vi "Update FIFO Address - 16-bit Address.vi"(0 "address in":u16, 5 "increment":bool, 7 "fifo depth":T1=10 items=["4"=2, "8"=3, "16"=4, "32"=5, "64"=6, "128"=7, "256"=8, "512"=9, "1024"=10, "2048"=11, "4096"=12, "8192"=13, "16384"=14, "32768"=15, "65536"=16]) -> (4 "address out":u16)   [LabVIEW 2011, in "FIFO.lvlib"]
uses:
  <instrlib>/RF-RIO/FIFO/FIFO/FPGA/FIFO.lvlib
  <instrlib>/RF-RIO/FIFO/FIFO/FPGA/Private/FIFO Depth - 16-bit Address.ctl
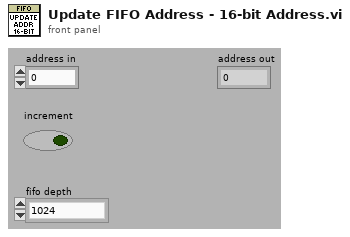
[diagram p1: front panel]
types:
  T1 = typedef "FIFO.lvlib/FIFO Depth - 16-bit Address.ctl" = u8
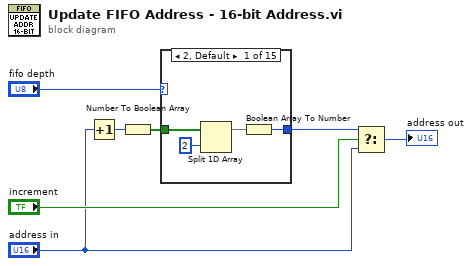
[diagram p0: block diagram]
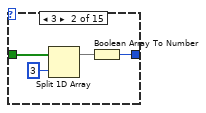
[diagram p2: hidden frame]
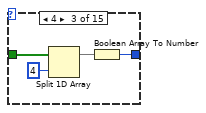
[diagram p3: hidden frame]
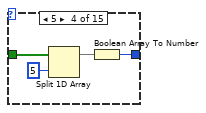
[diagram p4: hidden frame]
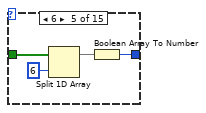
[diagram p5: hidden frame]
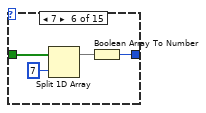
[diagram p6: hidden frame]
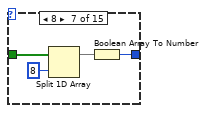
[diagram p7: hidden frame]
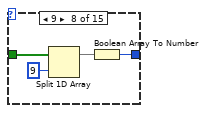
[diagram p8: hidden frame]
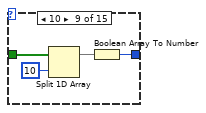
[diagram p9: hidden frame]
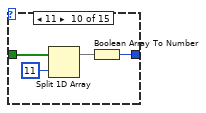
[diagram p10: hidden frame]
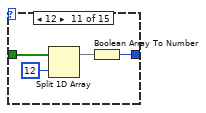
[diagram p11: hidden frame]
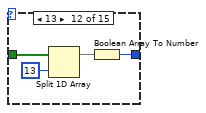
[diagram p12: hidden frame]
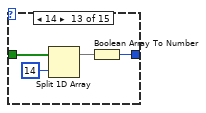
[diagram p13: hidden frame]
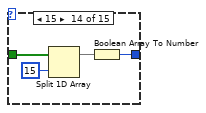
[diagram p14: hidden frame]
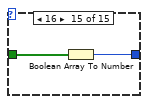
[diagram p15: hidden frame]
diagram:
  n1 = Increment(x="address in") -> (x+1=w2:u16)
  n2 = Number To Boolean Array(number=w2) -> (Boolean array=w1:bool[])
  n3 = case shown="2, Default" "fifo depth" {
    tunnel: w1 -> [w10 w14 w18 w22 w26 w30 w34 w38 w42 w46 w50 w54 w58 w62 w64]
    tunnel: [w11 w15 w19 w23 w27 w31 w35 w39 w43 w47 w51 w55 w59 w63 w65] -> w5
    frame 2, Default {
      n4 = Split 1D Array(array=w10, index=2) -> (first subarray=w8:bool[])  [unwired: 1 out]
      n5 = Boolean Array To Number(Boolean array=w8) -> (number=w11:u16)
    }
    frame 3 {
      n6 = Split 1D Array(array=w14, index=3) -> (first subarray=w12:bool[])  [unwired: 1 out]
      n7 = Boolean Array To Number(Boolean array=w12) -> (number=w15:u16)
    }
    frame 4 {
      n8 = Split 1D Array(array=w18, index=4) -> (first subarray=w16:bool[])  [unwired: 1 out]
      n9 = Boolean Array To Number(Boolean array=w16) -> (number=w19:u16)
    }
    frame 5 {
      n10 = Split 1D Array(array=w22, index=5) -> (first subarray=w20:bool[])  [unwired: 1 out]
      n11 = Boolean Array To Number(Boolean array=w20) -> (number=w23:u16)
    }
    frame 6 {
      n12 = Split 1D Array(array=w26, index=6) -> (first subarray=w24:bool[])  [unwired: 1 out]
      n13 = Boolean Array To Number(Boolean array=w24) -> (number=w27:u16)
    }
    frame 7 {
      n14 = Split 1D Array(array=w30, index=7) -> (first subarray=w28:bool[])  [unwired: 1 out]
      n15 = Boolean Array To Number(Boolean array=w28) -> (number=w31:u16)
    }
    frame 8 {
      n16 = Split 1D Array(array=w34, index=8) -> (first subarray=w32:bool[])  [unwired: 1 out]
      n17 = Boolean Array To Number(Boolean array=w32) -> (number=w35:u16)
    }
    frame 9 {
      n18 = Split 1D Array(array=w38, index=9) -> (first subarray=w36:bool[])  [unwired: 1 out]
      n19 = Boolean Array To Number(Boolean array=w36) -> (number=w39:u16)
    }
    frame 10 {
      n20 = Split 1D Array(array=w42, index=10) -> (first subarray=w40:bool[])  [unwired: 1 out]
      n21 = Boolean Array To Number(Boolean array=w40) -> (number=w43:u16)
    }
    frame 11 {
      n22 = Split 1D Array(array=w46, index=11) -> (first subarray=w44:bool[])  [unwired: 1 out]
      n23 = Boolean Array To Number(Boolean array=w44) -> (number=w47:u16)
    }
    frame 12 {
      n24 = Split 1D Array(array=w50, index=12) -> (first subarray=w48:bool[])  [unwired: 1 out]
      n25 = Boolean Array To Number(Boolean array=w48) -> (number=w51:u16)
    }
    frame 13 {
      n26 = Split 1D Array(array=w54, index=13) -> (first subarray=w52:bool[])  [unwired: 1 out]
      n27 = Boolean Array To Number(Boolean array=w52) -> (number=w55:u16)
    }
    frame 14 {
      n28 = Split 1D Array(array=w58, index=14) -> (first subarray=w56:bool[])  [unwired: 1 out]
      n29 = Boolean Array To Number(Boolean array=w56) -> (number=w59:u16)
    }
    frame 15 {
      n30 = Split 1D Array(array=w62, index=15) -> (first subarray=w60:bool[])  [unwired: 1 out]
      n31 = Boolean Array To Number(Boolean array=w60) -> (number=w63:u16)
    }
    frame 16 {
      n32 = Boolean Array To Number(Boolean array=w64) -> (number=w65:u16)
    }
  }
  n33 = Select(t=w5, s="increment", f="address in") -> (s? t:f=→"address out":u16)
